vi "Dashboard Main.vi"() -> ()   [LabVIEW 2013]
uses:
  <vilib>/event_ctls.llb/eventvkey.ctl
  <vilib>/Rock Robotics/WPI/Dashboard/WPI_DashboardLogging Global.vi
  <vilib>/Utility/config.llb/Write Key (String).vi
  <vilib>/Utility/config.llb/Write Key (I32).vi
  <vilib>/Utility/config.llb/NI_LVConfig.lvlib
panel:
  out "Image Message":string="Timeout in Camera Communications"
  in  "Rec Mode":enum32{"Stop", "Record", "Playback"}(radio)
  in  "Dashboard Tab":T1(tab)
  in  "Camera Settings":T2={"Frame Rate"=30, "Compression"=30, "Size"=1} {"Frame Rate" scale=1.0..30.0; "Size" items=["640x480", "320x240", "160x120"]}
  out "MotorSliders R":cluster{"MotorSlide1":dbl, "MotorSlide2":dbl} {"MotorSlide2" scale=-1.0..1.0 scale format="%#_2e"; "MotorSlide1" scale=-1.0..1.0 scale format="%#_2e"}
  out "MotorChart R":cluster{"Numeric":dbl, "Numeric":dbl}(graph)
  out "MotorSliders L":T3 {"MotorSlide4 2" scale=0.0..14.0 scale format="%#_2e"; "MotorSlide2" scale=-1.0..1.0 scale format="%#_2e"; "MotorSlide1" scale=-1.0..1.0 scale format="%#_2e"}
  out "MotorChart L":T4(graph)
  out "JS1 Z":dbl(slide) scale=-1.0..1.0 scale format="%#_2e"
  out "Joystick 1":cluster{"X":dbl, "Y":dbl}[](graph)
  out "JS Buttons 1":T5
  out "JS2 Z":dbl(slide) scale=-1.0..1.0 scale format="%#_2e"
  out "Joystick 2":cluster{"X":dbl, "Y":dbl}[](graph)
  out "JS Buttons 2":T5
  out "Mode":T6(ring)=enum."Auto Disabled"
  out "Camera IP":string
  in  "DB Camera Config":bool
  out "fps":dbl format="%#.1g"
  out "Mbps":dbl format="%#.1g"
  out "Mbps 2":bool
  out "LED 1":bool
  in  "Compressor On/Off":bool
  in  "Grabber Pistons Extended":bool
  out "Are Grabber Pistons Extended":bool
  in  "Camera Pitch Control":dbl
  in  "Camera Rotation Control":dbl
  out "Is The Firing Pin Piston Extended":bool
  out "Are Mechanism Pistons Extended":bool
  in  "Firing Pin Piston Extended":bool
  in  "Mechanism Piston Extended":bool
  in  "Manual Mechanism Override":bool
  in  "Checkbox 2":bool
  in  "Checkbox 1":bool
  in  "Test Slider":dbl(slide) scale=0.0..100.0 scale format="%#_3g"
  in  "On/Off":bool caption="Solenoid"
  in  "Test Name":u16(ring) items=["Select the test to run...", "Example Test", "-------------------------------", "List of tests is built in robot code.", "Replace with your own automated tests."]
  in  "Test Tree":string(tree)
  in  "Motor":cluster{"Value":dbl, "Enable":bool} {"Value" scale=-1.0..1.0 scale format="%#_3g"}
  out "Progress":T7 {"Test Progress" scale=0.0..100.0}
  in  "Rev/Fwd":cluster{"Forward":bool, "Reverse":bool}
  in  "Test Ring":u16(ring) items=["Auto", "Fixed indoor", "Fixed outdoor 1", "Fixed outdoor 2", "Fixed fluorescent 1", "Fixed fluorescent 2", "Hold current"]
  in  "Listbox":i32(listbox)
  out "Tree":string(tree)
  out "Camera Image":T8(plugin-control)
  in  "Enable":bool
  # "Left"
  # "Front"
  # "Right"
  # "Battery"
  # "This tab is a great place for autonomous settings and validation.\nCustomize by placing controls and indicators here and name to\nmatch Dashboard Variables on robot."
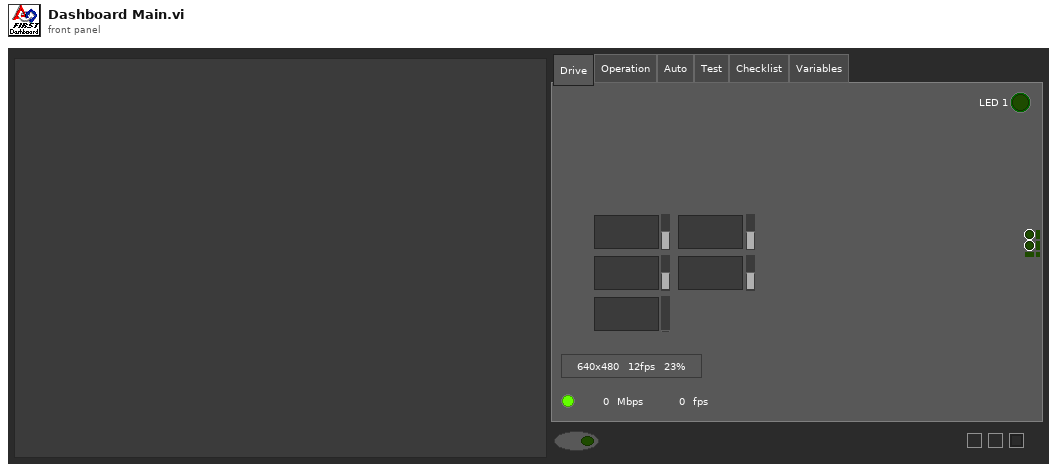
[diagram p1: front panel]
types:
  T1 = enum32{"Drive", "Operation", "Auto", "Test", "Checklist", "Variables"}
  T2 = cluster{"Frame Rate":i32, "Compression":i32, "Size":u16}
  T3 = cluster{"MotorSlide1":dbl, "MotorSlide2":dbl, "MotorSlide4 2":dbl}
  T4 = cluster{"Numeric":dbl, "Numeric":dbl, "Battery":sgl}
  T5 = cluster{bool, bool, bool, bool, bool, bool, bool, bool, bool, bool, bool, bool}
  T6 = enum8{"Tele-Op Disabled", "Tele-Op Enabled", "Auto Disabled", "Auto Enabled", "Test Disabled", "Test Enabled", ""}
  T7 = cluster{"Test Progress":u8, "Test Progress Text":string}
  T8 = typedef "IMAQ Image.ctl" = refnum<image>
  T9 = typedef "Image Type" = u32
  T10 = cluster{"Digital Inputs":bool[], "Digital Outputs":bool[]}
  T11 = cluster{"Competition mode":bool, "Robot Link":bool, "Autonomous":bool, "Enabled":bool, "E-Stop":bool, "Simulated":bool, "TestMode":bool, "Docked Window":bool}
  T12 = cluster{"Boolean Array[0]":bool, "Boolean Array[1]":bool, "Boolean Array[2]":bool, "Boolean Array[3]":bool, "Boolean Array[4]":bool, "Boolean Array[5]":bool, "Boolean Array[6]":bool, "Boolean Array[7]":bool, "Boolean Array[8]":bool, "Boolean Array[9]":bool, "Boolean Array[10]":bool, "Boolean Array[11]":bool}
  T13 = typedef "NI_LVConfig.lvlib/Config Data RefNum.ctl" = refnum<k1>
  T14 = typedef "eventvkey.ctl" = enum16{"ASCII", "Enter", "Return", "Shift", "Ctrl", "Alt", "Cmd", "Opt", "Caps", "NumLock", "Clear", "Break", "Up", "Down", "Left", "Right", "Insert", "Delete", "Home", "End", "PageUp", "PageDown", "Escape", "Help", "Pause", "ScrollLock", "F1", "F2", "F3", "F4", "F5", "F6", "F7", "F8", "F9", "F10", "F11", "F12", "F13", "F14", "F15", "F16", "F17", "F18", "F19", "F20", "F21", "F22", "F23", "F24", "Play", "VolumeUp", "VolumeDown", "Mute", "Two Byte Char"}
  T15 = cluster{"Image Size":bool, "Image Type":bool, "Pixel Value":bool, "ROI Information":bool, "Zoom Factor":bool}
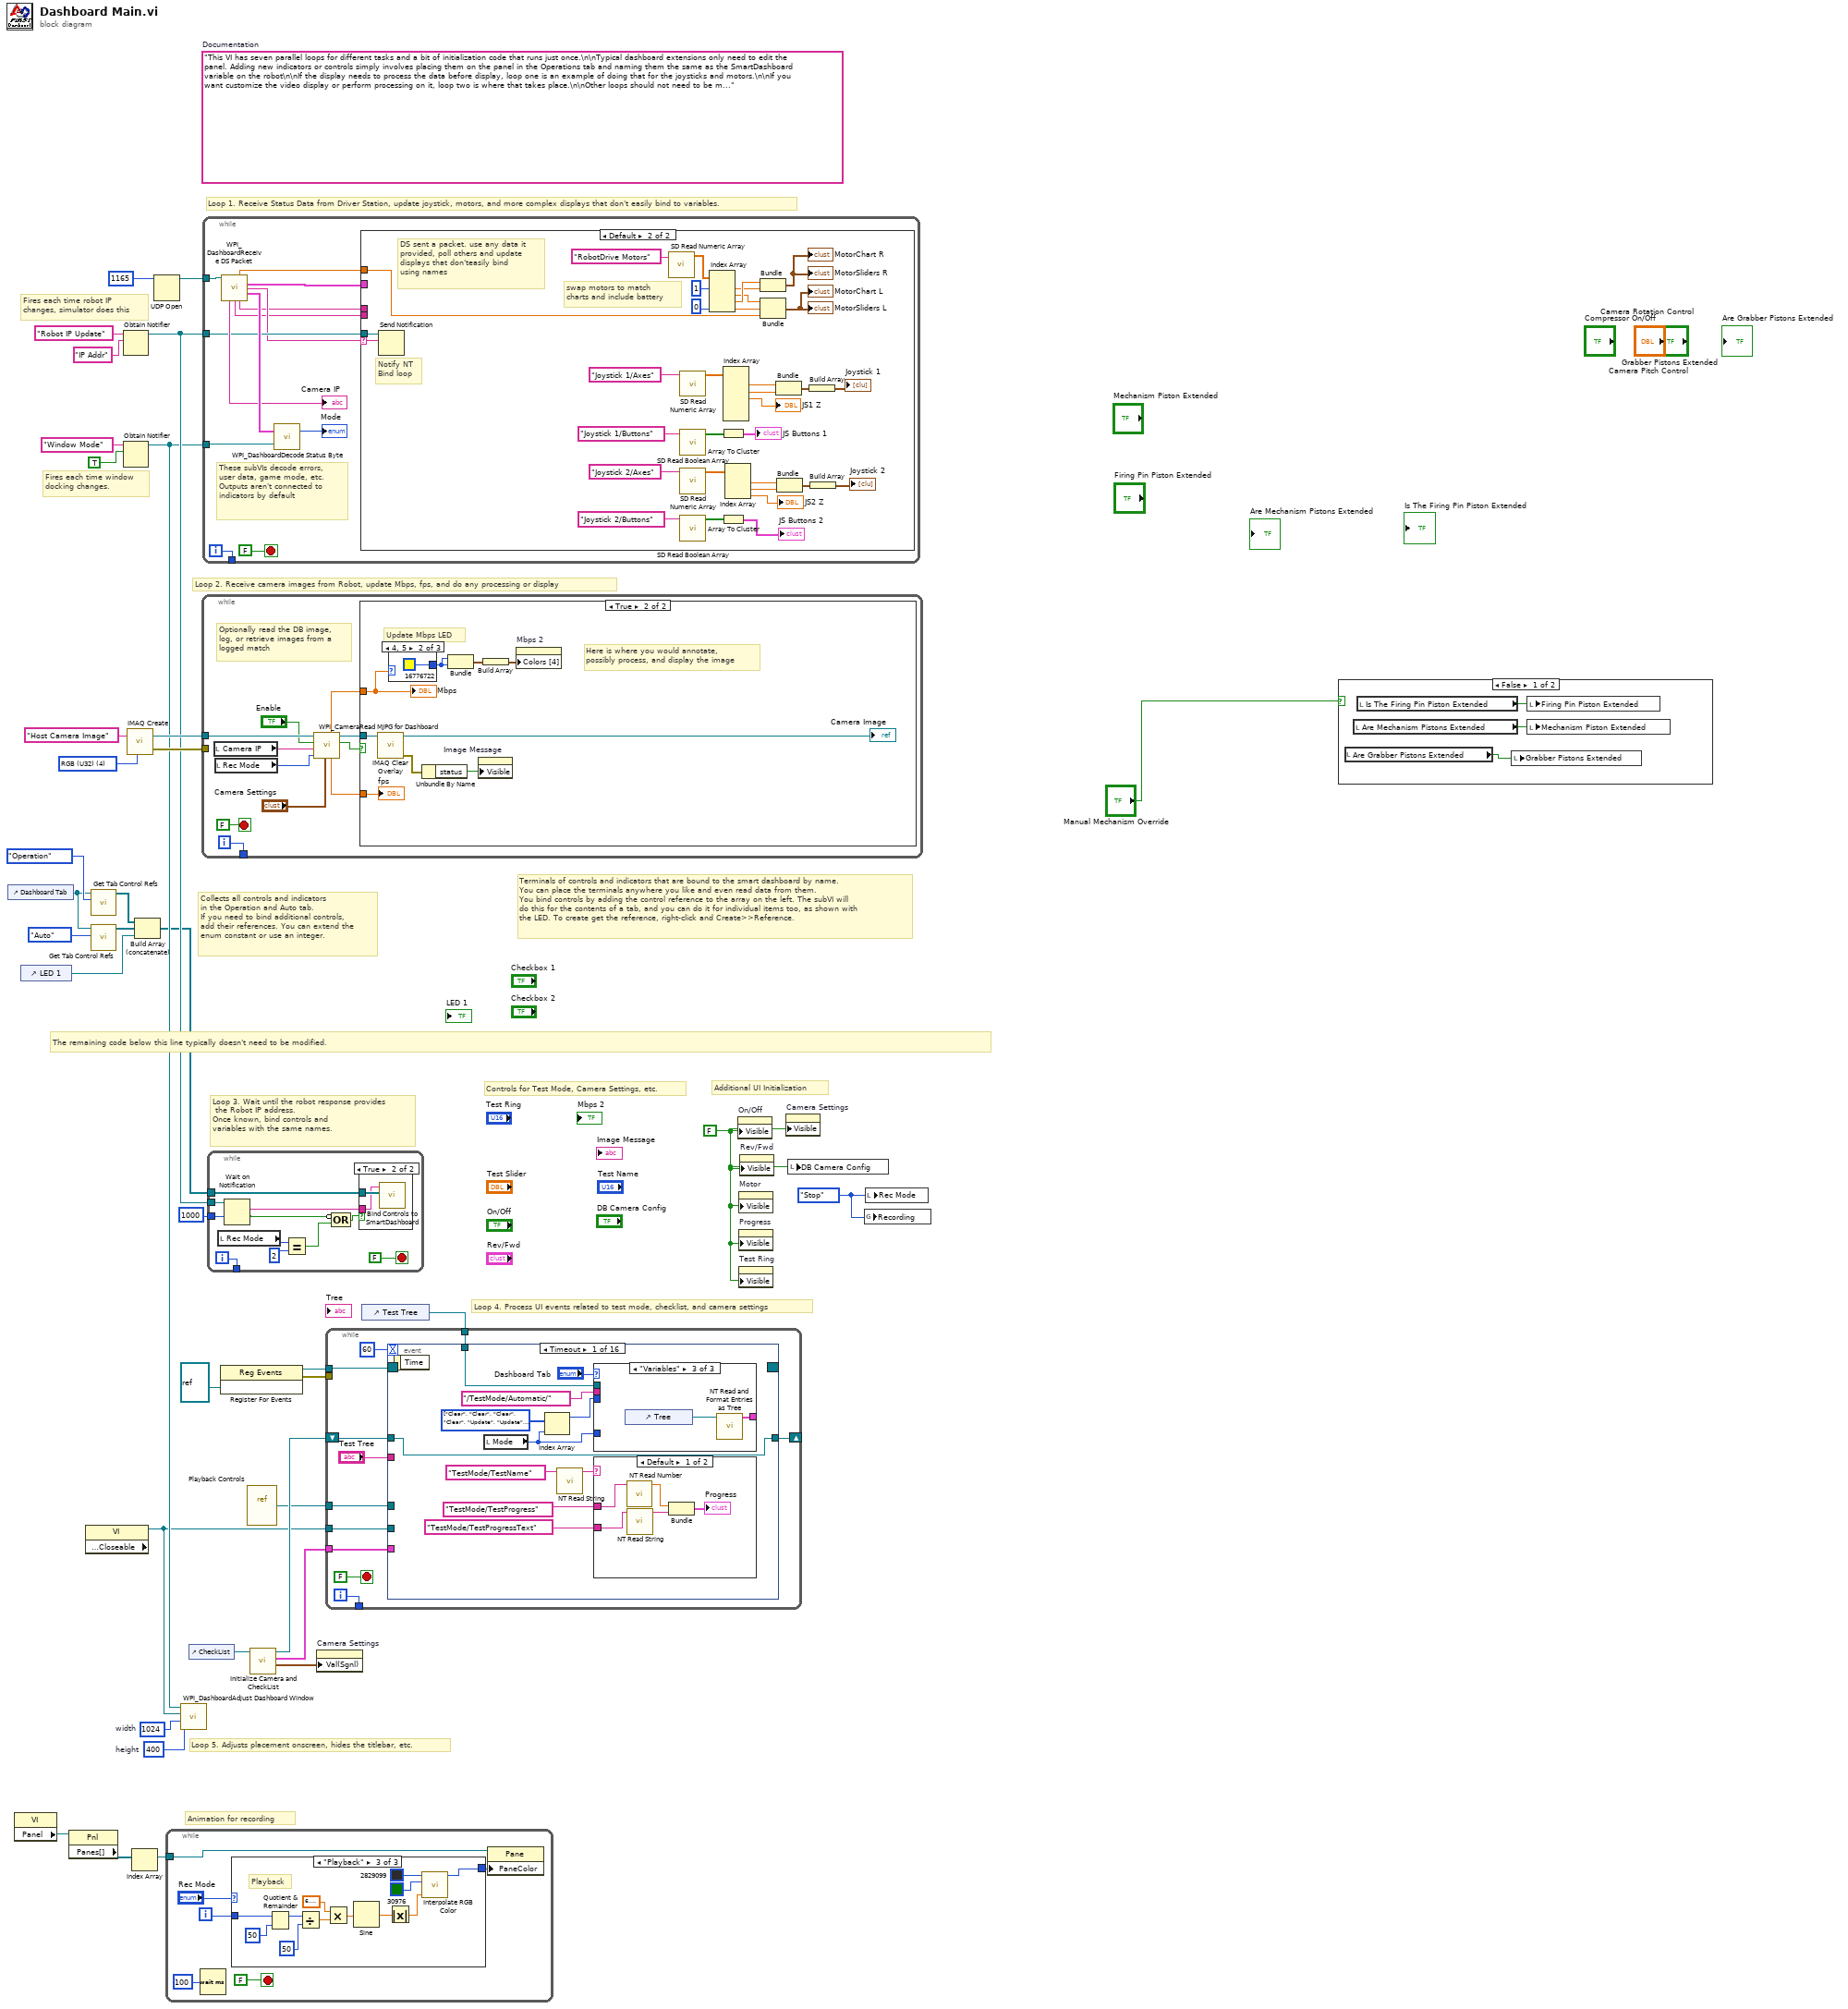
[diagram p0: block diagram]
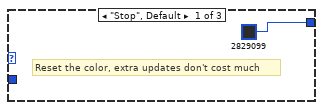
[diagram p3: hidden frame]
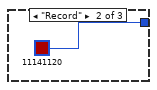
[diagram p4: hidden frame]
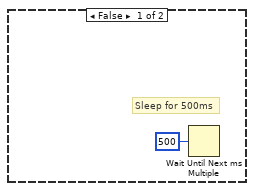
[diagram p6: hidden frame]
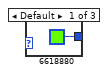
[diagram p7: hidden frame]
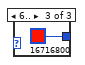
[diagram p8: hidden frame]
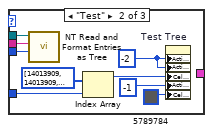
[diagram p10: hidden frame]
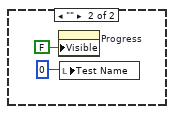
[diagram p11: hidden frame]
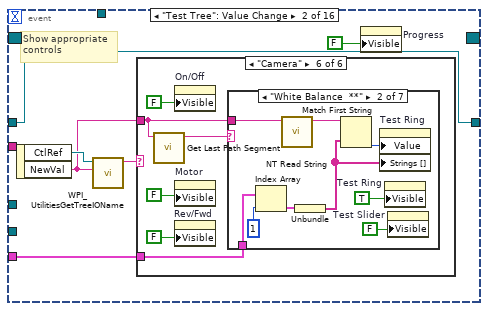
[diagram p12: hidden frame]
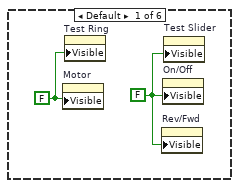
[diagram p13: hidden frame]
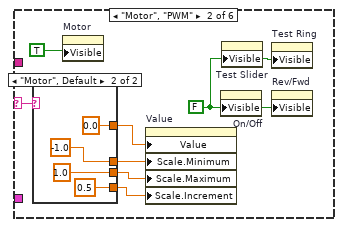
[diagram p14: hidden frame]
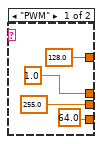
[diagram p15: hidden frame]
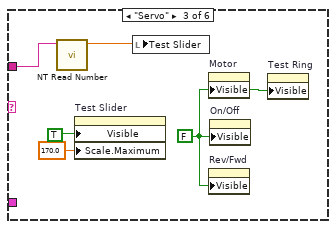
[diagram p16: hidden frame]
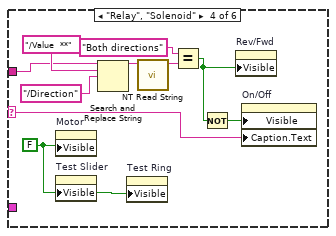
[diagram p17: hidden frame]
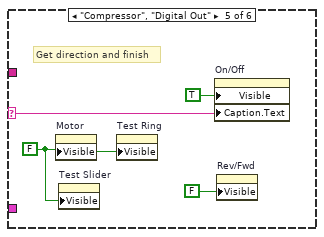
[diagram p18: hidden frame]
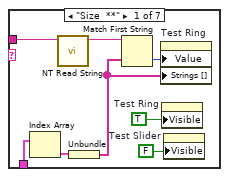
[diagram p19: hidden frame]
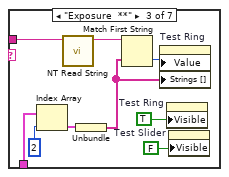
[diagram p20: hidden frame]
diagram:
  w9 = enum32{"Stop", "Record", "Playback"}."Stop" ("Rec Mode")
  w12 = 400  # height
  w13 = 1024  # width
  w26 = FALSE ("Visible")
  (unwired) "This VI has seven parallel loops for different tasks and a bit of initialization code that runs just once.\n\nTypical dashboard extensions only need to edit the panel. Adding new indicators or controls simply involves placing them on the panel in the Operations tab and naming them the same as the SmartDashboard variable on the robot\n\nIf the display needs to process the data before display, loop one is an example of doing that for the joysticks and motors.\n\nIf you want customize the video display or perform processing on it, loop two is where that takes place.\n\nOther loops should not need to be modified. They are pretty standard, and document the task they perform."  # Documentation
  w36 = T9 4 items=["Grayscale (U8)", "Grayscale (I16)", "Grayscale (SGL)", "Complex (CSG)", "RGB (U32)", "HSL (U32)", "RGB (U64)"] ("Image Type")
  # "Controls for Test Mode, Camera Settings, etc."
  # "Additional UI Initialization"
  # "Animation for recording"
  # "Fires each time robot IP\nchanges, simulator does this"
  # "Fires each time window\ndocking changes."
  # "Collects all controls and indicators\nin the Operation and Auto tab.\nIf you need to bind additional controls,\nadd their references. You can extend the\nenum constant or use an integer."
  # "The remaining code below this line typically doesn't need to be modified."
  # "Loop 4. Process UI events related to test mode, checklist, and camera settings"
  # "Terminals of controls and indicators that are bound to the smart dashboard by name.\nYou can place the terminals anywhere you like and even read data from them.\nYou bind controls by adding the control reference to the array on the left. The subVI will\ndo this for the contents of a tab, and you can do it for individual items too, as shown with\nthe LED. To create get the reference, right-click and Create>>Reference."
  # "Loop 3. Wait until the robot response provides\n the Robot IP address.\nOnce known, bind controls and\nvariables with the same names."
  # "Loop 5. Adjusts placement onscreen, hides the titlebar, etc."
  # "Loop 1. Receive Status Data from Driver Station, update joystick, motors, and more complex displays that don't easily bind to variables."
  # "Loop 2. Receive camera images from Robot, update Mbps, fps, and do any processing or display"
  n1 = control-ref of="Dashboard Tab"() -> (w7:refnum<vi>)
  n2 = property class="VI"() -> ("Panel"=w20:refnum<vi>)  [unwired: 2 in, 2 out]
  n3 = control-ref of="LED 1"() -> (w2:refnum<vi>)
  n4 = property class="Pnl"(reference=w20) -> ("Panes[]"=w21:refnum<vi>[])  [unwired: 1 in, 2 out]
  n5 = property class="VI" props=["Front Panel.Closeable"]() -> (reference out=w8:refnum<vi>)  [unwired: 2 in, 2 out]
  n6 = call <vilib>:"Get Tab Control Refs.vi"("Page Index"=T1."Operation" ("Dashboard Tab"), "TabControl in"=w7) -> ("ControlsOnPage"=w5:refnum<vi>[])  [unwired: 9 in]
  n7 = call <vilib>:"Get Tab Control Refs.vi"("Page Index"=T1."Auto" ("Dashboard Tab"), "TabControl in"=w7) -> ("ControlsOnPage"=w6:refnum<vi>[])  [unwired: 9 in]
  n8 = Obtain Notifier(name (unnamed)="Robot IP Update", notification data type="IP Addr" ("name (unnamed)")) -> (notifier out=w30:refnum<notifier>)  [unwired: 2 in, 2 out]
  n9 = Obtain Notifier(name (unnamed)="Window Mode", notification data type=TRUE) -> (notifier out=w11:refnum<notifier>)  [unwired: 2 in, 2 out]
  n10 = call "IMAQ Create"("Image Name"="Host Camera Image", "Image Type"=w36) -> ("New Image"=w34:T8, "error out"=w33:errorcluster)  [unwired: 2 in, 1 out]
  n11 = Index Array(array=w21) -> (element=w19:refnum<vi>)  [unwired: 1 in]
  n12 = Build Array (concatenate)(w5, w6, w2) -> (w4:refnum<vi>[])
  n13 = UDP Open(11:u16 1165 ("port")) -> (port=w37:refnum<k16>)  [unwired: 2 in, 4 out]
  n14 = while {
    tunnel: w19 -> [w40]
    i -> [w43]
    stop <- FALSE stop-if-true
    n15 = Wait (ms)(milliseconds to wait=u32 100) -> ()  [unwired: 1 out]
    n16 = case shown="\"Playback\"" "Rec Mode" {
      tunnel: w43 -> [_ _ w58]
      tunnel: [u32 2829099 ("Base Color") u32 11141120 ("Target Color") w47] -> w39
      frame "Stop", Default {
        # "Reset the color, extra updates don't cost much"
      }
      frame "Record" {
      }
      frame "Playback" {
        # "Playback"
        n17 = Quotient & Remainder(x=w58, y=u32 50 ("milliseconds to wait")) -> (x-y*floor(x/y)=w54:u32)  [unwired: 1 out]
        n18 = Divide(x=w54, y=u32 50 ("milliseconds to wait")) -> (x/y=w51:dbl)
        n19 = Multiply(x=6.283185307179586, y=w51) -> (x*y=w56:dbl)
        n20 = Sine(x=w56) -> (sin(x)=w55:dbl)
        n21 = Absolute Value(x=w55) -> (abs(x)=w48:dbl)
        n22 = call "Interpolate RGB Color.vi"("Proportion"=w48, "Target Color"=u32 30976, "Base Color"=u32 2829099) -> ("Result Color"=w47:u32)  [unwired: 8 in]
      }
    }
    n23 = property class="Pane"(reference=w40, "PaneColor"=w39) -> ()  [unwired: 1 in, 2 out]
  }
  n24 = call <vilib>:"WPI_DashboardAdjust Dashboard Window.vi"("height"=w12, "width"=w13, "reference in"=w8, "Notifier in"=w11) -> ()  [unwired: 8 in]
  n25 = control-ref of="CheckList"() -> (w10:refnum<vi>)
  n26 = while {
    tunnel: w34 -> [w67]
    tunnel: w33 -> [_]
    tunnel: [w68] -> _
    i -> [w68]
    stop <- FALSE stop-if-true
    # "Optionally read the DB image,\nlog, or retrieve images from a\nlogged match"
    n27 = local read "Camera IP"() -> (w60:string)
    n28 = local read "Rec Mode"() -> (w59:enum32{"Stop", "Record", "Playback"})
    n29 = call <vilib>:"WPI_CameraRead MJPG for Dashboard.vi"("Camera Settings"="Camera Settings", "Rec Mode"=w59, "Camera IP"=w60, "Enable"="Enable", "Refnum in"=w67) -> ("Active"=w64:bool, "Refnum out"=w66:T8, "FPS"=w63:dbl, "Bandwidth (Mbps)"=w62:dbl)  [unwired: 3 in]
    n30 = case shown="True" w64 {
      tunnel: w66 -> [_ w74]
      tunnel: w62 -> [_ w73]
      tunnel: w63 -> [_ w71]
      frame False {
        # "Sleep for 500ms"
        n31 = Wait Until Next ms Multiple(millisecond multiple=u32 500) -> ()  [unwired: 1 out]
      }
      frame True {
        # "Here is where you would annotate,\npossibly process, and display the image"
        # "Update Mbps LED"
        n32 = call "IMAQ Clear Overlay"("Image"=w74) -> ("error out"=w78:errorcluster, "Image Out"=→"Camera Image":T8)  [unwired: 2 in, 7 out]
        n33 = case shown="4, 5" w73 {
          tunnel: [u32 6618880 ("Color Box") u32 16776722 ("Color Box") u32 16716800 ("Color Box")] -> w75
          frame Default {
          }
          frame 4, 5 {
          }
          frame 6.. {
          }
        }
        n34 = Unbundle By Name(w78) -> ("status"=w79:bool)
        n35 = Bundle("Color Box"=w75, "Color Box"=w75) -> (w77:cluster{"Color Box":u32, "Color Box":u32})  [unwired: 1 out]
        n36 = property on="Image Message" class="Str"("Visible"=w79) -> ()  [unwired: 2 in, 2 out]
        n37 = Build Array(w77) -> (w76:cluster{"Color Box":u32, "Color Box":u32}[])
        n38 = property on="Mbps 2" class="Bool (strict)"("Colors [4]"=w76) -> ()  [unwired: 2 in, 2 out]
        "Mbps" <- w73
        "fps" <- w71
      }
    }
  }
  n39 = while {
    tunnel: w37 -> [w93]
    tunnel: w30 -> [w88]
    tunnel: w11 -> [w92]
    tunnel: [w89] -> _
    i -> [w89]
    stop <- FALSE stop-if-true
    # "These subVIs decode errors, user data, game mode, etc.\nOutputs aren't connected to indicators by default"
    n40 = call <vilib>:"WPI_DashboardReceive DS Packet.vi"("Recv Socket"=w93) -> ("Battery"=w83:sgl, "Driver Station"=w84:T10, "Robot IP Address"=w87:string, "Status"=w94:T11, "Camera IP Address"=→"Camera IP":string, "Low Priority User Data"=w86:string, "High Priority User Data"=w85:string)  [unwired: 1 in, 7 out]
    n41 = call <vilib>:"WPI_DashboardDecode Status Byte.vi"("Window Mode Notifier"=w92, "Status"=w94) -> ("Mode"=→"Mode":T6)  [unwired: 1 out]
    n42 = case shown="Default" w87 {
      selector: w87 -> [_ w106]
      tunnel: w88 -> [_ w107]
      tunnel: w86 -> [_ _]
      tunnel: w85 -> [_ _]
      tunnel: w84 -> [_ _]
      tunnel: w83 -> [_ w105]
      frame "0.0.0.0" {
        # "DS not sending packets, or no robot exists yet.\nDon't poll the variables"
      }
      frame Default {
        # "Notify NT\nBind loop"
        # "DS sent a packet. use any data it\nprovided, poll others and update\ndisplays that don'teasily bind\nusing names"
        # "swap motors to match\ncharts and include battery"
        n43 = Send Notification(notification=w106, notifier=w107) -> ()  [unwired: 1 in, 2 out]
        n44 = call <vilib>:"SD Read Numeric Array.vi"("Name"="RobotDrive Motors") -> ("Numeric Array"=w104:dbl[])  [unwired: 8 in, 2 out]
        n45 = call <vilib>:"SD Read Numeric Array.vi"("Name"="Joystick 1/Axes") -> ("Numeric Array"=w123:dbl[])  [unwired: 8 in, 2 out]
        n46 = call <vilib>:"SD Read Boolean Array.vi"("Name"="Joystick 1/Buttons") -> ("Boolean Array"=w125:bool[])  [unwired: 8 in, 2 out]
        n47 = call <vilib>:"SD Read Numeric Array.vi"("Name"="Joystick 2/Axes") -> ("Numeric Array"=w117:dbl[])  [unwired: 8 in, 2 out]
        n48 = call <vilib>:"SD Read Boolean Array.vi"("Name"="Joystick 2/Buttons") -> ("Boolean Array"=w116:bool[])  [unwired: 8 in, 2 out]
        n49 = Index Array(array=w104, index #1=1, index #4=0) -> (element #1=w100:dbl, element #2=w99:dbl, element #3=w101:dbl, element #4=w96:dbl)  [unwired: 2 in]
        n50 = Array To Cluster(array=w125) -> (cluster=→"JS Buttons 1":T12)
        n51 = Array To Cluster(array=w116) -> (cluster=→"JS Buttons 2":T12)
        n52 = Index Array(array=w123) -> (element #1=w120:dbl, element #2=w121:dbl, element #3=→"JS1 Z":dbl)  [unwired: 6 in, 3 out]
        n53 = Index Array(array=w117) -> (element #1=w112:dbl, element #2=w111:dbl, element #3=→"JS2 Z":dbl)  [unwired: 3 in]
        n54 = Bundle("Numeric"=w101, "Numeric"=w100) -> (→"MotorChart R" →"MotorSliders R":cluster{"Numeric":dbl, "Numeric":dbl})  [unwired: 1 in]
        n55 = Bundle("Numeric"=w99, "Numeric"=w96, "Battery"=w105) -> (→"MotorChart L" →"MotorSliders L":T4)  [unwired: 1 in]
        n56 = Bundle("Numeric"=w120, "Numeric"=w121) -> (w119:cluster{"Numeric":dbl, "Numeric":dbl})  [unwired: 1 in]
        n57 = Bundle("Numeric"=w112, "Numeric"=w111) -> (w113:cluster{"Numeric":dbl, "Numeric":dbl})  [unwired: 1 in]
        n58 = Build Array(w119) -> (→"Joystick 1":cluster{"Numeric":dbl, "Numeric":dbl}[])
        n59 = Build Array(w113) -> (→"Joystick 2":cluster{"Numeric":dbl, "Numeric":dbl}[])
      }
    }
  }
  n60 = while {
    tunnel: w4 -> [w139]
    tunnel: w30 -> [w137]
    tunnel: [w135] -> _
    tunnel: u32 1000 ("milliseconds to wait") -> [w134]
    i -> [w135]
    stop <- FALSE stop-if-true
    n61 = local read "Rec Mode"() -> (w130:enum32{"Stop", "Record", "Playback"})
    n62 = Wait on Notification(notifier=w137, timeout in ms (-1)=w134) -> (notification=w136:string, timed out?=w132:bool)  [unwired: 2 in, 2 out]
    n63 = Equal?(x=w130, y=u16 2 ("Rec Mode")) -> (x = y?=w131:bool)
    n64 = Compound Arithmetic op=OR(invert w132, w131) -> (w133:bool)
    n65 = case shown="True" w133 {
      tunnel: w139 -> [_ w141]
      tunnel: w136 -> [_ w140]
      frame False {
      }
      frame True {
        n66 = call <vilib>:"Bind Controls to SmartDashboard.vi"("Bound Control Refs"=w141, "Server IP Address"=w140) -> ()  [unwired: 10 in]
      }
    }
  }
  n67 = register-events(refnum<vi> refnum) -> (reference out=w17:refnum<event-registration>, error out=w16:errorcluster)  [unwired: 2 in]
  n68 = vi-ref "Playback Controls.vi"() -> (w18:refnum<vi>)
  n69 = call "Initialize Camera and CheckList.vi"("ListBox in"=w10) -> ("Cluster"=w24:cluster{"value":i32, "value":i32, "index":i32}, "Array"=w25:cluster{string[]}[], "File Refnum"=w23:T13)  [unwired: 8 in]
  n70 = property on="Camera Settings" class="Clust (strict)"("Val(Sgnl)"=w24) -> ()  [unwired: 2 in, 2 out]
  n71 = control-ref of="Test Tree"() -> (w22:refnum<vi>)
  n72 = while {
    tunnel: w25 -> [w149]
    shift-right: [w148] -> _
    shift-left: w23 -> [w147]
    tunnel: [w146] -> _
    tunnel: w22 -> [w145]
    tunnel: w18 -> [w144]
    tunnel: w17 -> [w143]
    tunnel: w16 -> [_]
    tunnel: w8 -> [w142]
    i -> [w146]
    stop <- FALSE stop-if-true
    n73 = event shown="[0] Timeout" {
      selector: w143 -> [_ _ _ _ _ _ _ _ _ _ _ _ _ _ _ _]
      dyn-events: [_ _ _ _ _ _ _ _ _ _ _ _ _ w387 _ _] -> _
      timeout: u32 60 ("milliseconds to wait") -> [_ _ _ _ _ _ _ _ _ _ _ _ _ _ _ _]
      tunnel: w145 -> [w159 _ _ _ _ _ _ _ _ _ _ _ _ _ _ _]
      tunnel: "Test Tree" -> [_ _ _ _ _ _ _ _ w356 w364 w366 w370 w378 _ _ _]
      tunnel: w149 -> [_ w183 _ _ _ _ w320 w350 _ _ _ _ _ _ _ _]
      tunnel: [w153 w182 w281 w286 w294 w306 w319 w343 w355 w362 w365 w369 w377 w389 w403 w404] -> w148
      tunnel: w147 -> [w153 w182 w281 w286 w294 w306 w318 w343 w355 w362 w365 w369 w377 w389 w403 w404]
      tunnel: w144 -> [_ _ _ _ _ _ _ _ _ _ _ _ _ w390 _ w407]
      tunnel: w142 -> [_ _ _ _ _ _ _ _ _ _ _ _ _ w385 _ _]
      event Timeout {
        w158 = enum16{"Update", "Clear"}[] [enum."Clear", enum."Clear", enum."Clear", enum."Clear", enum."Update", enum."Update", enum."Clear"] items=["Update", "Clear"]
        n74 = event-data() -> ()  [unwired: 1 in, 1 out]
        n75 = local read "Mode"() -> (w156:T6)
        n76 = Index Array(array=w158, index=w156) -> (element=w157:enum16{"Update", "Clear"})
        n77 = call <vilib>:"NT Read String.vi"("Name"="TestMode/TestName") -> ("String"=w162:string)  [unwired: 9 in, 1 out]
        n78 = case shown="\"Variables\"" "Dashboard Tab" {
          tunnel: w159 -> [_ w172 _]
          tunnel: "/TestMode/Automatic/" ("Name Pattern") -> [_ w171 _]
          tunnel: w157 -> [_ w170 _]
          tunnel: w156 -> [_ w168 _]
          tunnel: [_ _ w174] -> _
          frame "Operation", Default {
          }
          frame "Test" {
            w167 = -2 ("Active Item:Row Number")
            n79 = call <vilib>:"NT Read and Format Entries as Tree.vi"("Operation"=w170, "Name Pattern"=w171, "Tree Refnum"=w172) -> ()  [unwired: 7 in, 2 out]
            n80 = Index Array(array=u32[] [14013909, 14013909, 14013909, 14013909, 14013909, 16777215, 14013909], index=w168) -> (element=w166:u32)
            n81 = property on="Test Tree" class="Tree (strict)"("Active Item Row Number"=w167, "ActiveColNum"=w167, "CellBG"=w166, "Active Item Row Number"=-1 ("Active Item:Row Number"), "CellBG"=u32 5789784 ("Color Box")) -> ()  [unwired: 2 in, 2 out]
          }
          frame "Variables" {
            n82 = control-ref of="Tree"() -> (w173:refnum<vi>)
            n83 = call <vilib>:"NT Read and Format Entries as Tree.vi"("Tree Refnum"=w173) -> ("Formatted Strings"=w174:cluster{"Name":string, "Value":string}[])  [unwired: 9 in, 1 out]
          }
        }
        n84 = case shown="Default" w162 {
          tunnel: "TestMode/TestProgress" ("Name") -> [w176 _]
          tunnel: "TestMode/TestProgressText" ("Name") -> [w175 _]
          frame Default {
            n85 = call <vilib>:"NT Read Number.vi"("Name"=w176) -> ("Numeric"=w177:dbl)  [unwired: 9 in, 1 out]
            n86 = call <vilib>:"NT Read String.vi"("Name"=w175) -> ("String"=w178:string)  [unwired: 9 in, 1 out]
            n87 = Bundle("Numeric"=w177, "String"=w178) -> (→"Progress":cluster{"Numeric":dbl, "String":string})  [unwired: 1 in]
          }
          frame "" {
            n88 = property on="Progress" class="Clust (strict)"("Visible"=FALSE) -> ()  [unwired: 2 in, 2 out]
            n89 = local write "Test Name"(u16 0) -> ()
          }
        }
      }
      event "Test Tree": Value Change {
        # "Show appropriate\ncontrols"
        n90 = event-data() -> ("CtlRef"=w186:refnum<vi>, "NewVal"=w184:string)  [unwired: 1 in]
        n91 = call <vilib>:"WPI_UtilitiesGetTreeIOName.vi"("NewVal"=w184, "TreeControl in"=w186) -> ("I/O Name"=w187:string)  [unwired: 9 in]
        n92 = case shown="\"Camera\"" w187 {
          selector: w187 -> [_ w194 _ w212 w221 _]
          tunnel: w184 -> [_ _ w209 w211 _ w228]
          tunnel: w183 -> [_ _ _ _ _ w227]
          frame Default {
            w189 = FALSE ("Visible")
            w188 = FALSE ("Visible")
            n93 = property on="Motor" class="Clust (strict)"("Visible"=w188) -> ()  [unwired: 2 in, 2 out]
            n94 = property on="Test Ring" class="Ring (strict)"("Visible"=w188) -> ()  [unwired: 2 in, 2 out]
            n95 = property on="Rev/Fwd" class="Clust (strict)"("Visible"=w189) -> ()  [unwired: 2 in, 2 out]
            n96 = property on="On/Off" class="Bool (strict)"("Visible"=w189) -> ()  [unwired: 2 in, 2 out]
            n97 = property on="Test Slider" class="Slide (strict)"("Visible"=w189) -> ()  [unwired: 2 in, 2 out]
          }
          frame "Motor", "PWM" {
            w195 = FALSE ("Visible")
            n98 = case shown="\"Motor\", Default" w194 {
              tunnel: [1.0 ("Value") -1.0 ("Value")] -> w193
              tunnel: [255.0 ("Value") 1.0 ("Value")] -> w192
              tunnel: [128.0 ("Value") 0.0 ("Value")] -> w191
              tunnel: [64.0 ("Value") 0.5 ("Value")] -> w190
              frame "PWM" {
              }
              frame "Motor", Default {
              }
            }
            n99 = property on="Motor" class="Clust (strict)"("Visible"=TRUE) -> ()  [unwired: 2 in, 2 out]
            n100 = property on="Value" class="Slide (strict)"("Value"=w191, "Scale.Minimum"=w193, "Scale.Maximum"=w192, "Scale.Increment"=w190) -> ()  [unwired: 2 in, 2 out]
            n101 = property on="On/Off" class="Bool (strict)"("Visible"=w195) -> ()  [unwired: 2 in, 2 out]
            n102 = property on="Test Slider" class="Slide (strict)"("Visible"=w195) -> ()  [unwired: 2 in, 2 out]
            n103 = property on="Test Ring" class="Ring (strict)"("Visible"=w195) -> ()  [unwired: 2 in, 2 out]
            n104 = property on="Rev/Fwd" class="Clust (strict)"("Visible"=w195) -> ()  [unwired: 2 in, 2 out]
          }
          frame "Servo" {
            w207 = FALSE ("Visible")
            n105 = call <vilib>:"NT Read Number.vi"("Name"=w209) -> ("Numeric"=w208:dbl)  [unwired: 9 in, 1 out]
            n106 = property on="Test Slider" class="Slide (strict)"("Visible"=TRUE, "Scale.Maximum"=170.0 ("Scale.Range:Maximum")) -> ()  [unwired: 2 in, 2 out]
            n107 = local write "Test Slider"(w208) -> ()
            n108 = property on="Motor" class="Clust (strict)"("Visible"=w207) -> ()  [unwired: 2 in, 2 out]
            n109 = property on="Rev/Fwd" class="Clust (strict)"("Visible"=w207) -> ()  [unwired: 2 in, 2 out]
            n110 = property on="On/Off" class="Bool (strict)"("Visible"=w207) -> ()  [unwired: 2 in, 2 out]
            n111 = property on="Test Ring" class="Ring (strict)"("Visible"=w207) -> ()  [unwired: 2 in, 2 out]
          }
          frame "Relay", "Solenoid" {
            w210 = FALSE ("Visible")
            n112 = property on="Motor" class="Clust (strict)"("Visible"=w210) -> ()  [unwired: 2 in, 2 out]
            n113 = property on="Test Slider" class="Slide (strict)"("Visible"=w210) -> ()  [unwired: 2 in, 2 out]
            n114 = Search and Replace String(input string=w211, search string="/Value  **", replace string="/Direction") -> (result string=w217:string)  [unwired: 5 in, 3 out]
            n115 = property on="Test Ring" class="Ring (strict)"("Visible"=w210) -> ()  [unwired: 2 in, 2 out]
            n116 = call <vilib>:"NT Read String.vi"("Name"=w217) -> ("String"=w215:string)  [unwired: 9 in, 1 out]
            n117 = Equal?(x="Both directions", y=w215) -> (x = y?=w213:bool)
            n118 = Not(x=w213) -> (.not. x?=w214:bool)
            n119 = property on="Rev/Fwd" class="Clust (strict)"("Visible"=w213) -> ()  [unwired: 2 in, 2 out]
            n120 = property on="On/Off" class="Bool (strict)"("Visible"=w214, "Caption.Text"=w212) -> ()  [unwired: 2 in, 2 out]
          }
          frame "Compressor", "Digital Out" {
            w220 = FALSE ("Visible")
            # "Get direction and finish"
            n121 = property on="Motor" class="Clust (strict)"("Visible"=w220) -> ()  [unwired: 2 in, 2 out]
            n122 = property on="Test Slider" class="Slide (strict)"("Visible"=w220) -> ()  [unwired: 2 in, 2 out]
            n123 = property on="Test Ring" class="Ring (strict)"("Visible"=w220) -> ()  [unwired: 2 in, 2 out]
            n124 = property on="On/Off" class="Bool (strict)"("Visible"=TRUE, "Caption.Text"=w221) -> ()  [unwired: 2 in, 2 out]
            n125 = property on="Rev/Fwd" class="Clust (strict)"("Visible"=FALSE) -> ()  [unwired: 2 in, 2 out]
          }
          frame "Camera" {
            n126 = call <vilib>:"Get Last Path Segment.vi"("String in"=w228) -> ("String out"=w229:string)  [unwired: 10 in]
            n127 = property on="On/Off" class="Bool (strict)"("Visible"=FALSE) -> ()  [unwired: 2 in, 2 out]
            n128 = property on="Motor" class="Clust (strict)"("Visible"=FALSE) -> ()  [unwired: 2 in, 2 out]
            n129 = property on="Rev/Fwd" class="Clust (strict)"("Visible"=FALSE) -> ()  [unwired: 2 in, 2 out]
            n130 = case shown="\"White Balance  **\"" w229 {
              tunnel: w228 -> [w235 w244 w253 w262 w271 _ w277]
              tunnel: w227 -> [w233 w241 w250 w259 w268 _ _]
              frame "Size  **" {
                n131 = Index Array(array=w233) -> (element=w232:cluster{string[]})  [unwired: 1 in]
                n132 = call <vilib>:"NT Read String.vi"("Name"=w235) -> ("String"=w234:string)  [unwired: 9 in, 1 out]
                n133 = Unbundle(w232) -> (w230:string[])
                n134 = Match First String(2:w230, 3:w234) -> (0:w231:i32)  [unwired: 1 out]
                n135 = property on="Test Ring" class="Ring (strict)"("Value"=w231, "Strings []"=w230) -> ()  [unwired: 2 in, 2 out]
                n136 = property on="Test Ring" class="Ring (strict)"("Visible"=TRUE) -> ()  [unwired: 2 in, 2 out]
                n137 = property on="Test Slider" class="Slide (strict)"("Visible"=FALSE) -> ()  [unwired: 2 in, 2 out]
              }
              frame "White Balance  **" {
                n138 = Index Array(array=w241, index=1) -> (element=w242:cluster{string[]})
                n139 = call <vilib>:"NT Read String.vi"("Name"=w244) -> ("String"=w243:string)  [unwired: 9 in, 1 out]
                n140 = Unbundle(w242) -> (w239:string[])
                n141 = Match First String(2:w239, 3:w243) -> (0:w238:i32)  [unwired: 1 out]
                n142 = property on="Test Ring" class="Ring (strict)"("Value"=w238, "Strings []"=w239) -> ()  [unwired: 2 in, 2 out]
                n143 = property on="Test Ring" class="Ring (strict)"("Visible"=TRUE) -> ()  [unwired: 2 in, 2 out]
                n144 = property on="Test Slider" class="Slide (strict)"("Visible"=FALSE) -> ()  [unwired: 2 in, 2 out]
              }
              frame "Exposure  **" {
                n145 = Index Array(array=w250, index=2) -> (element=w251:cluster{string[]})
                n146 = call <vilib>:"NT Read String.vi"("Name"=w253) -> ("String"=w252:string)  [unwired: 9 in, 1 out]
                n147 = Unbundle(w251) -> (w247:string[])
                n148 = Match First String(2:w247, 3:w252) -> (0:w248:i32)  [unwired: 1 out]
                n149 = property on="Test Ring" class="Ring (strict)"("Value"=w248, "Strings []"=w247) -> ()  [unwired: 2 in, 2 out]
                n150 = property on="Test Ring" class="Ring (strict)"("Visible"=TRUE) -> ()  [unwired: 2 in, 2 out]
                n151 = property on="Test Slider" class="Slide (strict)"("Visible"=FALSE) -> ()  [unwired: 2 in, 2 out]
              }
              frame "Exposure Priority  **" {
                n152 = Index Array(array=w259, index=3) -> (element=w260:cluster{string[]})
                n153 = call <vilib>:"NT Read String.vi"("Name"=w262) -> ("String"=w261:string)  [unwired: 9 in, 1 out]
                n154 = Unbundle(w260) -> (w256:string[])
                n155 = Match First String(2:w256, 3:w261) -> (0:w257:i32)  [unwired: 1 out]
                n156 = property on="Test Ring" class="Ring (strict)"("Value"=w257, "Strings []"=w256) -> ()  [unwired: 2 in, 2 out]
                n157 = property on="Test Ring" class="Ring (strict)"("Visible"=TRUE) -> ()  [unwired: 2 in, 2 out]
                n158 = property on="Test Slider" class="Slide (strict)"("Visible"=FALSE) -> ()  [unwired: 2 in, 2 out]
              }
              frame "Color Enable  **" {
                n159 = Index Array(array=w268, index=4) -> (element=w269:cluster{string[]})
                n160 = call <vilib>:"NT Read String.vi"("Name"=w271) -> ("String"=w270:string)  [unwired: 9 in, 1 out]
                n161 = Unbundle(w269) -> (w265:string[])
                n162 = Match First String(2:w265, 3:w270) -> (0:w266:i32)  [unwired: 1 out]
                n163 = property on="Test Ring" class="Ring (strict)"("Value"=w266, "Strings []"=w265) -> ()  [unwired: 2 in, 2 out]
                n164 = property on="Test Ring" class="Ring (strict)"("Visible"=TRUE) -> ()  [unwired: 2 in, 2 out]
                n165 = property on="Test Slider" class="Slide (strict)"("Visible"=FALSE) -> ()  [unwired: 2 in, 2 out]
              }
              frame Default {
                n166 = property on="Test Ring" class="Ring (strict)"("Visible"=FALSE) -> ()  [unwired: 2 in, 2 out]
                n167 = property on="Test Slider" class="Slide (strict)"("Visible"=FALSE) -> ()  [unwired: 2 in, 2 out]
              }
              frame "Brightness  **", "Color Level  **", "Compression  **", "FPS  **", "Sharpness  **" {
                n168 = call <vilib>:"NT Read Number.vi"("Name"=w277) -> ("Numeric"=w276:dbl)  [unwired: 9 in, 1 out]
                n169 = local write "Test Slider"(w276) -> ()
                n170 = property on="Test Slider" class="Slide (strict)"("Visible"=TRUE, "Scale.Maximum"=100.0 ("Scale.Range:Maximum")) -> ()  [unwired: 2 in, 2 out]
                n171 = property on="Test Ring" class="Ring (strict)"("Visible"=FALSE) -> ()  [unwired: 2 in, 2 out]
              }
            }
          }
        }
        n172 = property on="Progress" class="Clust (strict)"("Visible"=FALSE) -> ()  [unwired: 2 in, 2 out]
      }
      event "Test Name": Mouse Enter {
        # "Populate the ring with the list of tests"
        n173 = event-data() -> ()  [unwired: 1 in, 1 out]
        n174 = call <vilib>:"NT Read String Array.vi"("Name"="TestMode/TestList") -> ("String Array"=w285:string[])  [unwired: 9 in, 1 out]
        n175 = Build Array (concatenate)("Select the test to run...", w285) -> (w284:string[])
        n176 = property on="Test Name" class="Ring (strict)"("Strings []"=w284) -> ()  [unwired: 2 in, 2 out]
      }
      event "Test Name": Value Change {
        w287 = FALSE ("Visible")
        # "Tell the robot the test name to run"
        n177 = event-data() -> ("NewVal"=w291:u16)  [unwired: 1 in]
        n178 = property on="Test Name" class="Ring (strict)"() -> ("Strings []"=w292:string[])  [unwired: 2 in, 2 out]
        n179 = local write "Progress"(T7 {"Test Progress"=0, "Test Progress Text"=""} ("Progress")) -> ()
        n180 = Index Array(array=w292, index=w291) -> (element=w290:string)
        n181 = call <vilib>:"NT Write String.vi"("String"=w290, "Name"="TestMode/TestName") -> ()  [unwired: 9 in, 1 out]
        n182 = property on="Progress" class="Clust (strict)"("Visible"=TRUE) -> ()  [unwired: 2 in, 2 out]
        n183 = property on="Motor" class="Clust (strict)"("Visible"=w287) -> ()  [unwired: 2 in, 2 out]
        n184 = property on="Test Slider" class="Slide (strict)"("Visible"=w287) -> ()  [unwired: 2 in, 2 out]
        n185 = property on="On/Off" class="Bool (strict)"("Visible"=w287) -> ()  [unwired: 2 in, 2 out]
        n186 = property on="Rev/Fwd" class="Clust (strict)"("Visible"=w287) -> ()  [unwired: 2 in, 2 out]
        n187 = property on="Test Ring" class="Ring (strict)"("Visible"=w287) -> ()  [unwired: 2 in, 2 out]
      }
      event "Listbox": Double Click {
        n188 = event-data() -> ("PlatMods.Shift"=w295:bool, "Row"=w297:i32)  [unwired: 1 in]
        n189 = case shown="True" w295 {
          tunnel: w297 -> [w301 _]
          tunnel: 1 -> [w300 _]
          frame False {
            n190 = property on="Listbox" class="LstBox (strict)"() -> ("Item Symbols"=w299:i32[])  [unwired: 2 in, 2 out]
            n191 = Replace Array Subset(array=w299, new element=w300, index=w301) -> (w298:i32[])
            n192 = property on="Listbox" class="LstBox (strict)"("Item Symbols"=w298) -> ()  [unwired: 2 in, 2 out]
          }
          frame True {
            w302 = 0 ("Top Row")
            n193 = property on="Listbox" class="LstBox (strict)"() -> ("Number of Rows"=w304:u32)  [unwired: 2 in, 2 out]
            n194 = Initialize Array(0, w304) -> (w303:i32[])
            n195 = property on="Listbox" class="LstBox (strict)"("Top Row"=w302, "Value"=w302, "Item Symbols"=w303) -> ()  [unwired: 2 in, 2 out]
          }
        }
      }
      event "Listbox": Key Down {
        n196 = event-data() -> ("VKey"=w308:T14)  [unwired: 1 in]
        n197 = case shown="\"Left\", \"Right\"" w308 {
          selector: w308 -> [w313 _]
          tunnel: eventvkey."Left" ("VKey") -> [w311 _]
          frame "Left", "Right" {
            n198 = Equal?(x=w311, y=w313) -> (x = y?=w312:bool)
            n199 = Select(t=0, s=w312, f=1) -> (s? t:f=w314:i32)
            n200 = property on="Listbox" class="LstBox (strict)"() -> ("Item Symbols"=w317:i32[])  [unwired: 2 in, 2 out]
            n201 = Replace Array Subset(array=w317, new element=w314, index="Listbox") -> (w316:i32[])
            n202 = property on="Listbox" class="LstBox (strict)"("Item Symbols"=w316) -> ()  [unwired: 2 in, 2 out]
          }
          frame Default {
          }
        }
      }
      event "DB Camera Config": Value Change {
        n203 = event-data() -> ("NewVal"=w321:bool)  [unwired: 1 in]
        n204 = case shown="False" w321 {
          tunnel: w320 -> [w330 _]
          tunnel: [w323 w341] -> w319
          tunnel: w318 -> [w322 w341]
          frame False {
            w337 = "Camera"
            w340 = FALSE ("Visible")
            n205 = local read "Camera Settings"() -> (w329:T2)
            n206 = Index Array(array=w330) -> (element=w333:cluster{string[]})  [unwired: 1 in]
            n207 = Unbundle(w329) -> ("Frame Rate"=w328:i32, "Compression"=w327:i32, "Size"=w331:u16)
            n208 = Unbundle(w333) -> (w332:string[])
            n209 = Index Array(array=w332, index=w331) -> (element=w326:string)
            n210 = call-poly <vilib>:"Write Key.vi"("section"=w337, "value"=w326, "key"="Size", "refnum"=w322) -> ("refnum out"=w339:T13)  [unwired: 2 in, 5 out]
            n211 = call-poly <vilib>:"Write Key.vi"("section"=w337, "value"=w328, "key"="FrameRate", "refnum"=w339) -> ("refnum out"=w338:T13)  [unwired: 1 in, 6 out]
            n212 = property on="Camera Settings" class="Clust (strict)"("Visible"=w340) -> ()  [unwired: 2 in, 2 out]
            n213 = local write "DB Camera Config"(w340) -> ()
            n214 = call-poly <vilib>:"Write Key.vi"("section"=w337, "value"=w327, "key"="Compression", "refnum"=w338) -> ("refnum out"=w324:T13)  [unwired: 1 in, 6 out]
            n215 = call <vilib>:"Close Config Data.vi"("refnum"=w324) -> ("file path"=w325:path)  [unwired: 2 in, 8 out]
            n216 = call <vilib>:"Open Config Data.vi"("configuration file path"=w325) -> ("refnum"=w323:T13)  [unwired: 8 in, 2 out]
          }
          frame True {
            n217 = property on="Camera Settings" class="Clust (strict)"("Visible"=TRUE) -> ()  [unwired: 2 in, 2 out]
          }
        }
      }
      event "Camera Settings": Value Change {
        n218 = event-data() -> ("NewVal"=w354:T2)  [unwired: 1 in]
        n219 = Index Array(array=w350) -> (element=w349:cluster{string[]})  [unwired: 1 in]
        n220 = Unbundle(w354) -> ("Frame Rate"=w345:i32, "Compression"=w344:i32, "Size"=w347:u16)
        n221 = Unbundle(w349) -> (w348:string[])
        n222 = Index Array(array=w348, index=w347) -> (element=w346:string)
        n223 = Format Into String(format string="%s   %dfps   %d%%", w346, w345, w344) -> (resulting string=w351:string)  [unwired: 2 in, 1 out]
        n224 = Build Array(w351) -> (w352:string[])
        n225 = property on="DB Camera Config" class="Bool (strict)"("Strings [4]"=w352) -> ()  [unwired: 2 in, 2 out]
      }
      event "Motor.Enable": Value Change {
        n226 = event-data() -> ("NewVal"=w360:bool)  [unwired: 1 in]
        n227 = Unbundle("Motor") -> ("Value"=w359:dbl)  [unwired: 1 out]
        n228 = Select(t=w359, s=w360, f=0.0) -> (s? t:f=w357:dbl)
        n229 = call <vilib>:"NT Write Number.vi"("Numeric"=w357, "Name"=w356) -> ()  [unwired: 9 in, 1 out]
      }
      event "Test Slider": Value Change {
        n230 = event-data() -> ("NewVal"=w363:dbl)  [unwired: 1 in]
        n231 = call <vilib>:"NT Write Number.vi"("Numeric"=w363, "Name"=w364) -> ()  [unwired: 9 in, 1 out]
      }
      event "On/Off": Value Change {
        n232 = event-data() -> ("NewVal"=w368:bool)  [unwired: 1 in]
        n233 = Boolean To (0,1)(Boolean=w368) -> (0, 1=w367:i16)
        n234 = call <vilib>:"NT Write Number.vi"("Numeric"=w367, "Name"=w366) -> ()  [unwired: 9 in, 1 out]
      }
      event "Rev/Fwd": Value Change {
        n235 = event-data() -> ("NewVal.Forward"=w376:bool, "NewVal.Reverse"=w375:bool)  [unwired: 1 in]
        n236 = Boolean To (0,1)(Boolean=w376) -> (0, 1=w372:i16)
        n237 = Boolean To (0,1)(Boolean=w375) -> (0, 1=w374:i16)
        n238 = Negate(x=w374) -> (-x=w373:i16)
        n239 = Add(x=w372, y=w373) -> (x+y=w371:i16)
        n240 = call <vilib>:"NT Write Number.vi"("Numeric"=w371, "Name"=w370) -> ()  [unwired: 9 in, 1 out]
      }
      event "Test Ring": Value Change {
        n241 = event-data() -> ("NewVal"=w380:u16)  [unwired: 1 in]
        n242 = property on="Test Ring" class="Ring (strict)"() -> ("Strings []"=w381:string[])  [unwired: 2 in, 2 out]
        n243 = Index Array(array=w381, index=w380) -> (element=w379:string)
        n244 = call <vilib>:"NT Write String.vi"("String"=w379, "Name"=w378) -> ()  [unwired: 9 in, 1 out]
      }
      event "Rec Mode": Value Change {
        # "Update globals for recording mode and path to read log from.\nClear when logging and let NetworkTables set path for vision to\nuse."
        n245 = event-data() -> ("NewVal"=w391:enum32{"Stop", "Record", "Playback"})  [unwired: 1 in]
        n246 = global write "WPI_DashboardLogging Global.vi" "Logging Filename"(path "") -> ()
        n247 = case shown="\"Stop\", \"Record\"" w391 {
          tunnel: w390 -> [_ w393 w401]
          tunnel: [_ _ w400] -> w387
          tunnel: [_ _ w399] -> _
          tunnel: w385 -> [_ _ w397]
          tunnel: cluster{i32, i32} {-250, 170} -> [_ _ w396]
          tunnel: [_ _ T15 {"Image Size"=TRUE, "Image Type"=TRUE, "Pixel Value"=TRUE, "ROI Information"=TRUE, "Zoom Factor"=FALSE} ("Image Information Shown:All Elements")] -> w383
          tunnel: [_ _ TRUE ("Zoom Factor")] -> w382
          frame Default {
          }
          frame "Stop", "Record" {
            # "Place Window too"
            n248 = invoke class="VI" method="FP.Close"(reference=w393) -> (reference out=w392:refnum<vi>)  [unwired: 2 in, 2 out]
            n249 = invoke class="VI" method="Abort VI"(reference=w392) -> ()  [unwired: 2 in, 3 out]
          }
          frame "Playback" {
            n250 = call "Open Playback Panel.vi"("Offset"=w396, "DB VI Ref"=w397, "Playback in"=w401) -> ("Playback out"=w398:refnum<vi>)  [unwired: 8 in]
            n251 = register-events(w398) -> (reference out=w400:refnum<event-registration>, error out=w399:errorcluster)  [unwired: 2 in]
          }
        }
        n252 = global write "WPI_DashboardLogging Global.vi" "Recording"(w391) -> ()
        n253 = property on="Camera Image" class="ImageControl"("Image Information Shown"=w383, "Image Information Visible"=w382) -> ()  [unwired: 2 in, 2 out]
        n254 = call <vilib>:"WPI_DashboardNT Log FieldName Cache.vi"("Operation"=enum16{"Lookup/Add", "Index", "Clear"}."Clear") -> ()  [unwired: 8 in, 3 out]
      }
      event Panel Close {
        w402 = enum32{"Stop", "Record", "Playback"}."Stop" ("Rec Mode")
        n255 = event-data() -> ()  [unwired: 1 in, 4 out]
        n256 = local write "Rec Mode"(w402) -> ()
        n257 = global write "WPI_DashboardLogging Global.vi" "Recording"(w402) -> ()
      }
      event Panel Close {
        # "Abort playback window and ourself"
        n258 = event-data() -> ()  [unwired: 1 in, 4 out]
        n259 = invoke class="VI" method="FP.Close"(reference=w407) -> (reference out=w406:refnum<vi>)  [unwired: 2 in, 2 out]
        n260 = invoke class="VI" method="Abort VI"(reference=w406) -> (error out=w405:errorcluster)  [unwired: 2 in, 2 out]
        n261 = invoke class="VI" method="Abort VI"(error in=w405) -> ()  [unwired: 2 in, 3 out]
      }
    }
  }
  n262 = property on="On/Off" class="Bool (strict)"("Visible"=w26) -> ()  [unwired: 2 in, 2 out]
  n263 = property on="Motor" class="Clust (strict)"("Visible"=w26) -> ()  [unwired: 2 in, 2 out]
  n264 = property on="Progress" class="Clust (strict)"("Visible"=w26) -> ()  [unwired: 2 in, 2 out]
  n265 = property on="Test Ring" class="Ring (strict)"("Visible"=w26) -> ()  [unwired: 2 in, 2 out]
  n266 = property on="Rev/Fwd" class="Clust (strict)"("Visible"=w26) -> ()  [unwired: 2 in, 2 out]
  n267 = property on="Camera Settings" class="Clust (strict)"("Visible"=w26) -> ()  [unwired: 2 in, 2 out]
  n268 = local write "DB Camera Config"(w26) -> ()
  n269 = global write "WPI_DashboardLogging Global.vi" "Recording"(w9) -> ()
  n270 = local write "Rec Mode"(w9) -> ()
  n271 = case shown="False" "Manual Mechanism Override" {
    frame False {
      n272 = local read "Are Grabber Pistons Extended"() -> (w408:bool)
      n273 = local read "Are Mechanism Pistons Extended"() -> (w409:bool)
      n274 = local read "Is The Firing Pin Piston Extended"() -> (w410:bool)
      n275 = local write "Grabber Pistons Extended"(w408) -> ()
      n276 = local write "Firing Pin Piston Extended"(w410) -> ()
      n277 = local write "Mechanism Piston Extended"(w409) -> ()
    }
    frame True {
    }
  }
